vi "OE1022_Configure Sample.vi"(7 "OE1022_Configure Sample":T1={"Trigger Mode"=0, "Sample Mode"=0, "Buffer 1"=0, "Buffer 2"=1, "Buffer 3"=2, "Sample Time(ms)"=100, "Length"=50, "Buffer 4"=3, "Sample State"=2} {"Sample State" items=["Start", "Pause", "Stop and Clear"]; "Buffer 4" items=["R", "X", "Y", "Theta", "Rh1", "Xh1", "Yh1", "Theta h1", "Rh2", "Xh2", "Yh2", "Theta h2", "Noise", "A1", "A2", "A3", "A4", "E1", "E2", "E3", "E4", "Freq"]; "Length" min=1 max=16384; "Sample Time(ms)" min=1 max=100000; "Buffer 3" items=["R", "X", "Y", "Theta", "Rh1", "Xh1", "Yh1", "Theta h1", "Rh2", "Xh2", "Yh2", "Theta h2", "Noise", "A1", "A2", "A3", "A4", "E1", "E2", "E3", "E4", "Freq"]; "Buffer 2" items=["R", "X", "Y", "Theta", "Rh1", "Xh1", "Yh1", "Theta h1", "Rh2", "Xh2", "Yh2", "Theta h2", "Noise", "A1", "A2", "A3", "A4", "E1", "E2", "E3", "E4", "Freq"]; "Buffer 1" items=["R", "X", "Y", "Theta", "Rh1", "Xh1", "Yh1", "Theta h1", "Rh2", "Xh2", "Yh2", "Theta h2", "Noise", "A1", "A2", "A3", "A4", "E1", "E2", "E3", "E4", "Freq"]; "Sample Mode" items=["Single", "Loop"]; "Trigger Mode" items=["Int", "Ext"]}, 8 "Error in (no error)":errorcluster caption="error out（no error）", 9 "Remote Mode":u16(ring) items=["USB"=0, "GPIB"=2], 11 "VISA resource name":refnum<visa-resource-name>) -> (0 "Error out":errorcluster caption="error out", 1 "Output String":string, 3 "VISA resource  out":refnum<visa-resource-name>)   [LabVIEW 2011]
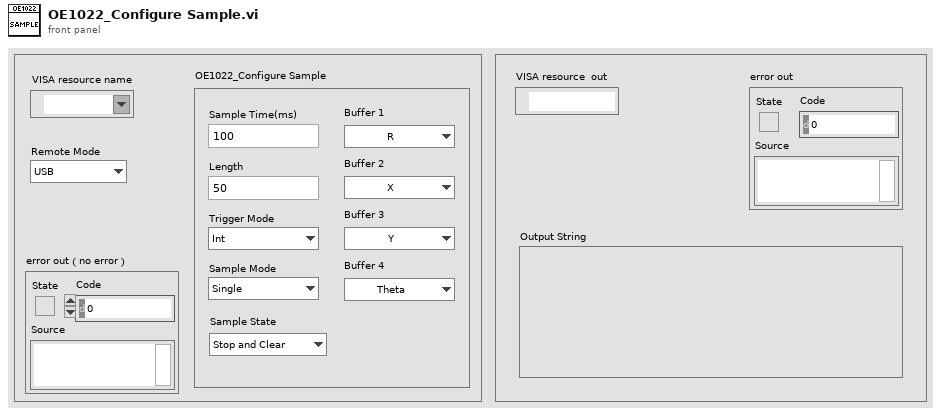
[diagram p1: front panel]
types:
  T1 = cluster{"Trigger Mode":u16, "Sample Mode":u16, "Buffer 1":u16, "Buffer 2":u16, "Buffer 3":u16, "Sample Time(ms)":u32, "Length":u16, "Buffer 4":u16, "Sample State":u16}
  T2 = enum16{"ISRC", "IGND", "ICPL", "ILIN", "PHAS", "FMOD", "RSLP", "FREQ", "SWPT", "SLLM", "SULM", "SSLL", "SSLG", "STLM", "SWRM", "IRNG", "SENS", "RMOD", "OFLT", "OFSL", "SYNC", "DMOD", "HARM", "DARB", "SWVT", "SLVL", "SVLL", "SVUL", "SVSL", "SVSG", "SVTM", "SVRM", "RALL", "SNAP", "OUTP", "OAUX", "COUT", "CAUX", "COFP", "CEXP", "FPOP", "OEXP", "*IDN", "*RST", "OVLD", "INOV", "GNOV", "*PLL", "SSET", "RSET", "AGAN", "APHS", "ARSV", "ASCL", "EQCD", "EQCS", "SPED", "SRAT", "SLEN", "SSLE", "STRG", "SPRM", "STRD", "PAUS", "REST", "SPTS", "TRCA", "TEMP", "RSTU", "IHNZ", "DEQU", "SADD", "ARNG", "CSPE", "ISRCD", "IGNDD", "ICPLD", "ILIND", "PHASD", "FMODD", "RSLPD", "FREQD", "SWPTD", "SLLMD", "SULMD", "SSLLD", "SSLGD", "STLMD", "SWRMD", "SENSD", "RMODD", "OFLTD", "OFSLD", "SYNCD", "HARMD", "EQCDD", "EQCSD", "SNAPD", "OUTPD", "SWVTD", "SLVLD", "SVLLD", "SVULD", "SVSLD", "SVSGD", "SVTMD", "SVRMD", "SVDCD", "ARSVD", "AGAND", "APHSD", "ASCLD", "FPOPD", "CAUXD", "OEXPD", "SPEDD", "SRATD", "SLEND", "SSLED", "STRGD", "SPRMD", "STRDD", "PAUSD", "RESTD", "SPTSD", "TRCAD", "*IDND", "*RSTD", "INOVD", "GNOVD", "*PLLD", "SSETD", "RSETD"}
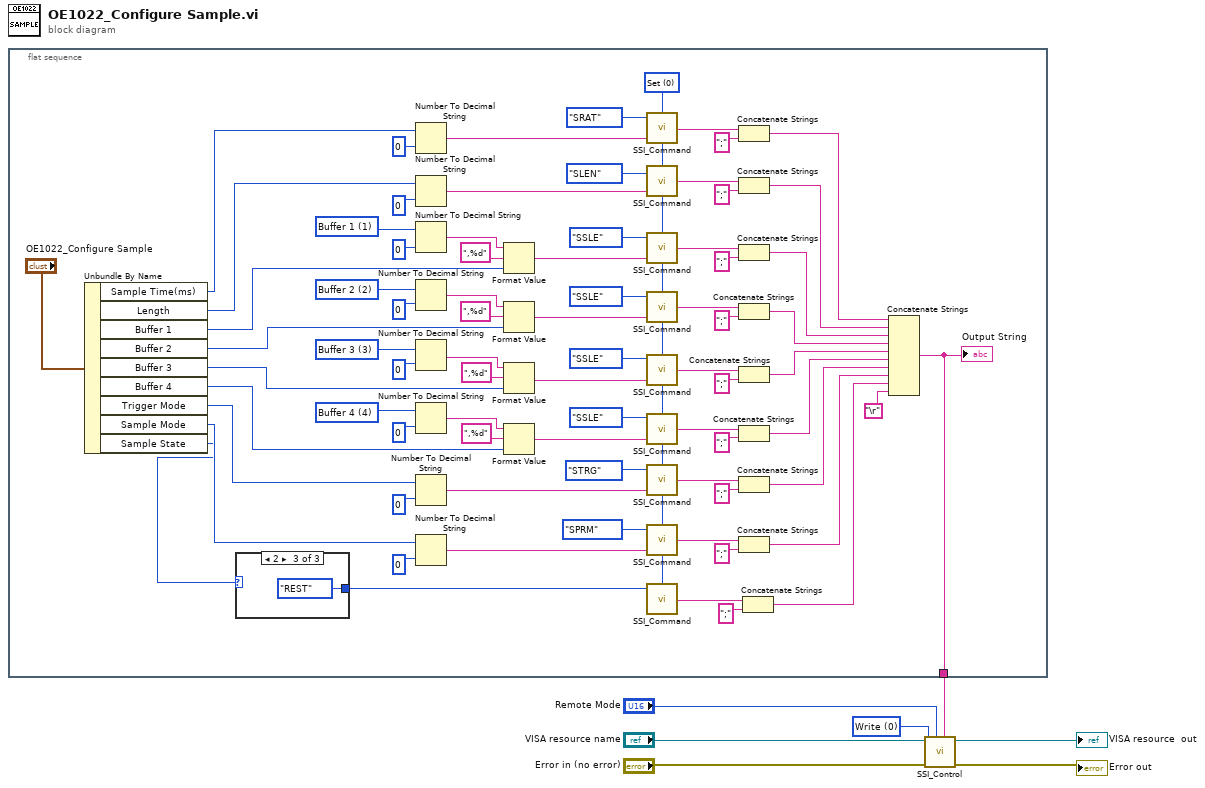
[diagram p0: block diagram]
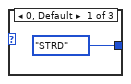
[diagram p2: hidden frame]
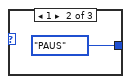
[diagram p3: hidden frame]
diagram:
  w6 = u16 0 items=["Write", "Read"] ("Control")
  n1 = flat-sequence {
    tunnel: [w82] -> w1
    frame #0 {
      w47 = u16 4 items=["Buffer 1"=1, "Buffer 2"=2, "Buffer 3"=3, "Buffer 4"=4]
      w54 = u16 3 items=["Buffer 1"=1, "Buffer 2"=2, "Buffer 3"=3, "Buffer 4"=4]
      w59 = u16 2 items=["Buffer 1"=1, "Buffer 2"=2, "Buffer 3"=3, "Buffer 4"=4]
      w8 = u16 0 items=["Set", "Query"] ("Opera")
      w64 = u16 1 items=["Buffer 1"=1, "Buffer 2"=2, "Buffer 3"=3, "Buffer 4"=4]
      n2 = Unbundle By Name("OE1022_Configure Sample") -> ("Sample Time(ms)"=w15:u32, "Length"=w16:u16, "Buffer 1"=w62:u16, "Buffer 2"=w58:u16, "Buffer 3"=w53:u16, "Buffer 4"=w48:u16, "Trigger Mode"=w51:u16, "Sample Mode"=w52:u16, "Sample State"=w14:u16)
      n3 = case shown="2" w14 {
        tunnel: [T2."STRD" ("Command Type") T2."PAUS" ("Command Type") T2."REST" ("Command Type")] -> w13
        frame 0, Default {
        }
        frame 1 {
        }
        frame 2 {
        }
      }
      n4 = Number To Decimal String(number=w15, width (-)=i16 0 ("精度(6)")) -> (decimal integer string=w68:string)
      n5 = Number To Decimal String(number=w16, width (-)=i16 0 ("宽度(-)")) -> (decimal integer string=w67:string)
      n6 = Number To Decimal String(number=w64, width (-)=i16 0 ("宽度(-)")) -> (decimal integer string=w63:string)
      n7 = Number To Decimal String(number=w59, width (-)=i16 0 ("宽度(-)")) -> (decimal integer string=w60:string)
      n8 = Number To Decimal String(number=w54, width (-)=i16 0 ("宽度(-)")) -> (decimal integer string=w55:string)
      n9 = Number To Decimal String(number=w47, width (-)=i16 0 ("宽度(-)")) -> (decimal integer string=w46:string)
      n10 = Number To Decimal String(number=w51, width (-)=i16 0 ("宽度(-)")) -> (decimal integer string=w41:string)
      n11 = Number To Decimal String(number=w52, width (-)=i16 0 ("宽度(-)")) -> (decimal integer string=w42:string)
      n12 = Format Value(string ("")=w63, format string=",%d" ("格式字符串"), value (0)=w62) -> (output string=w65:string)
      n13 = Format Value(string ("")=w60, format string=",%d" ("格式字符串"), value (0)=w58) -> (output string=w45:string)
      n14 = Format Value(string ("")=w55, format string=",%d" ("格式字符串"), value (0)=w53) -> (output string=w44:string)
      n15 = Format Value(string ("")=w46, format string=",%d" ("格式字符串"), value (0)=w48) -> (output string=w43:string)
      n16 = call "SSI_Command.vi"("Opera"=w8, "Paramter"=w68, "Command Type"=T2."SRAT") -> ("Output string"=w40:string)  [unwired: 1 in]
      n17 = call "SSI_Command.vi"("Opera"=w8, "Paramter"=w67, "Command Type"=T2."SLEN") -> ("Output string"=w35:string)  [unwired: 1 in]
      n18 = call "SSI_Command.vi"("Opera"=w8, "Paramter"=w65, "Command Type"=T2."SSLE") -> ("Output string"=w36:string)  [unwired: 1 in]
      n19 = call "SSI_Command.vi"("Opera"=w8, "Paramter"=w45, "Command Type"=T2."SSLE") -> ("Output string"=w34:string)  [unwired: 1 in]
      n20 = call "SSI_Command.vi"("Opera"=w8, "Paramter"=w44, "Command Type"=T2."SSLE") -> ("Output string"=w32:string)  [unwired: 1 in]
      n21 = call "SSI_Command.vi"("Opera"=w8, "Paramter"=w43, "Command Type"=T2."SSLE") -> ("Output string"=w30:string)  [unwired: 1 in]
      n22 = call "SSI_Command.vi"("Opera"=w8, "Paramter"=w41, "Command Type"=T2."STRG") -> ("Output string"=w28:string)  [unwired: 1 in]
      n23 = call "SSI_Command.vi"("Opera"=w8, "Paramter"=w42, "Command Type"=T2."SPRM") -> ("Output string"=w26:string)  [unwired: 1 in]
      n24 = call "SSI_Command.vi"("Opera"=w8, "Command Type"=w13) -> ("Output string"=w11:string)  [unwired: 2 in]
      n25 = Concatenate Strings(w40, ";" ("替换字符串(\"\")")) -> (w24:string)
      n26 = Concatenate Strings(w35, ";" ("替换字符串(\"\")")) -> (w23:string)
      n27 = Concatenate Strings(w36, ";" ("替换字符串(\"\")")) -> (w22:string)
      n28 = Concatenate Strings(w34, ";" ("替换字符串(\"\")")) -> (w21:string)
      n29 = Concatenate Strings(w32, ";" ("替换字符串(\"\")")) -> (w20:string)
      n30 = Concatenate Strings(w30, ";" ("替换字符串(\"\")")) -> (w19:string)
      n31 = Concatenate Strings(w28, ";" ("替换字符串(\"\")")) -> (w18:string)
      n32 = Concatenate Strings(w26, ";" ("替换字符串(\"\")")) -> (w17:string)
      n33 = Concatenate Strings(w11, ";" ("替换字符串(\"\")")) -> (w10:string)
      n34 = Concatenate Strings(w24, w23, w22, w21, w20, w19, w18, w17, w10, "\r") -> (w82:string)
      "Output String" <- w82
    }
  }
  n35 = call "SSI_Control.vi"("Write Buffer"=w1, "Remote Mode"="Remote Mode", "Error in (no error)"="Error in (no error)", "Control"=w6, "VISA resource name"="VISA resource name") -> ("Error out"=→"Error out":errorcluster, "VISA resource  out"=→"VISA resource  out":refnum<visa-resource-name>)  [unwired: 3 in, 2 out]
